vi "VIImageExport.vi"() -> ()   [LabVIEW 8.6]
panel:
  in  "VIPanelSavePath":path
  in  "OPEN":bool
  in  "JPEG file":path
  out "2D Picture":picture
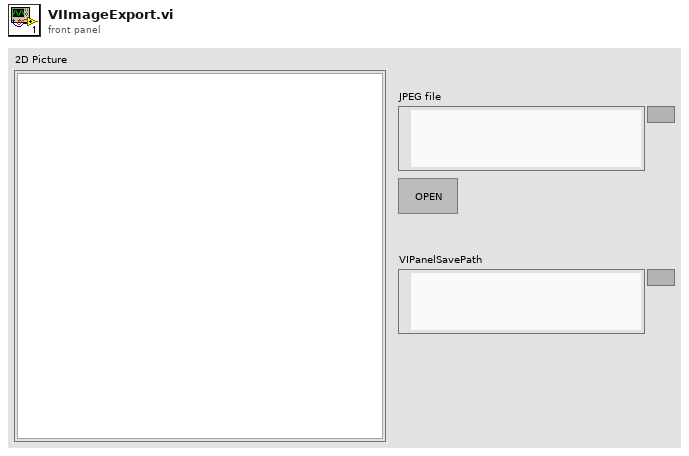
[diagram p1: front panel]
types:
  T1 = typedef "imagedata.ctl" = cluster{"image type":i32, "image depth":i32, "image":u8[], "mask":u8[], "colors":u32[], "Rectangle":cluster{"left":i16, "top":i16, "right":i16, "bottom":i16}}
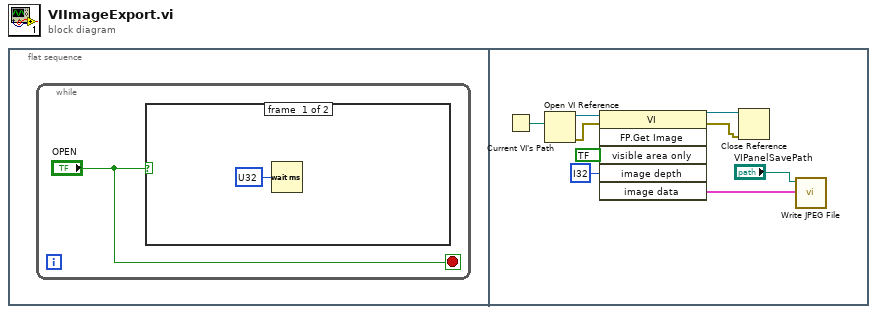
[diagram p0: block diagram]
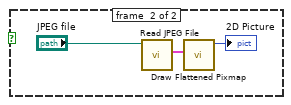
[diagram p2: hidden frame]
diagram:
  n1 = flat-sequence {
    frame #0 {
      n2 = while {
        stop <- "OPEN" stop-if-true
        n3 = case shown="True" "OPEN" {
          frame #0 {
            n4 = Wait (ms)(milliseconds to wait=u32 ?) -> ()  [unwired: 1 out]
          }
          frame #1 {
            n5 = call <vilib>:"Read JPEG File.vi"("path to JPEG file"="JPEG file") -> ("image data"=w5:T1)  [unwired: 8 in, 2 out]
            n6 = call <vilib>:"Draw Flattened Pixmap.vi"("image data"=w5) -> ("new picture"=→"2D Picture":picture)  [unwired: 8 in]
          }
        }
      }
    }
    frame #1 {
      n7 = Current VI's Path() -> (path=w14:path)
      n8 = Open VI Reference(vi path=w14) -> (vi reference=w13:refnum<vi>, error out=w12:errorcluster)  [unwired: 5 in]
      n9 = invoke class="VI" method="FP.Get Image"(reference=w13, error in=w12, "visible area only"=bool ? ("Visible Area Only"), "image depth"=i32 ? ("Image Depth")) -> (reference out=w10:refnum<vi>, error out=w11:errorcluster, "image data"=w8:T1)  [unwired: 2 in, 3 out]
      n10 = Close Reference(reference=w10, error in (no error)=w11) -> ()  [unwired: 1 out]
      n11 = call <vilib>:"Write JPEG File.vi"("image data"=w8, "path to JPEG file"="VIPanelSavePath") -> ()  [unwired: 8 in, 2 out]
    }
  }
